vi "File.vi"() -> ()   [LabVIEW 2020]
panel:
  out "error out":errorcluster
  in  "error in":errorcluster
  in  "start path":path=path "D:/"
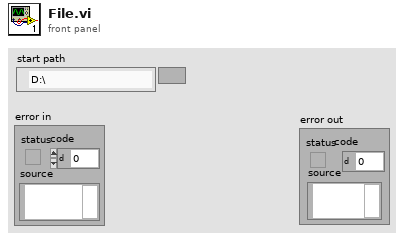
[diagram p1: front panel]
types:
  T1 = enum16{"open", "replace", "create", "open or create", "replace or create", "replace or create with confirmation"}
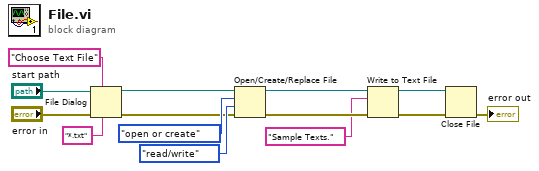
[diagram p0: block diagram]
diagram:
  n1 = File Dialog(6:"*.txt" ("pattern (all files)"), 7:"Choose Text File", 8:"error in", 11:"start path") -> (0:w4:errorcluster, 3:w5:path)  [unwired: 3 in, 2 out]
  n2 = Open/Create/Replace File(file path (use dialog)=w5, error in=w4, operation (0:open)=T1."open or create", access (0:read/write)=enum16{"read/write", "read-only", "write-only"}."read/write") -> (refnum out=w14:refnum<file>, error out=w12:errorcluster)  [unwired: 2 in, 1 out]
  n3 = Write to Text File(file (use dialog)=w14, text="Sample Texts.", error in=w12) -> (refnum out=w13:refnum<file>, error out=w11:errorcluster)  [unwired: 1 in, 1 out]
  n4 = Close File(refnum=w13, error in=w11) -> (error out=→"error out":errorcluster)  [unwired: 1 out]
